vi "epx_Vector_SC_Menu.vi"(8 "Run Mode?":bool, 11 "MenuRef":refnum<k9>) -> ()   [LabVIEW 2011, in "NI_EP_Basic.lvlib" / "EPX Vector Diagram.xctl"]
uses:
  <vilib>/addons/Electrical Power/Basic/Controls/Vector Diagram/EPX Vector Diagram.xctl
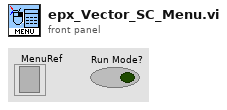
[diagram p1: front panel]
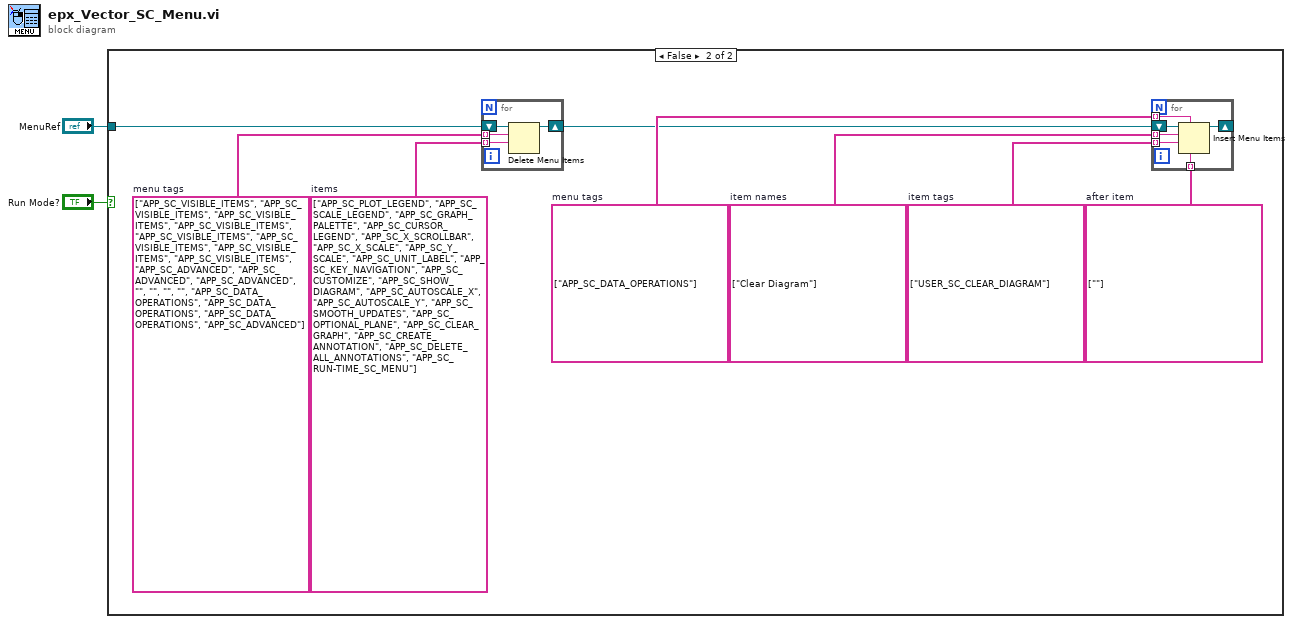
[diagram p0: block diagram]
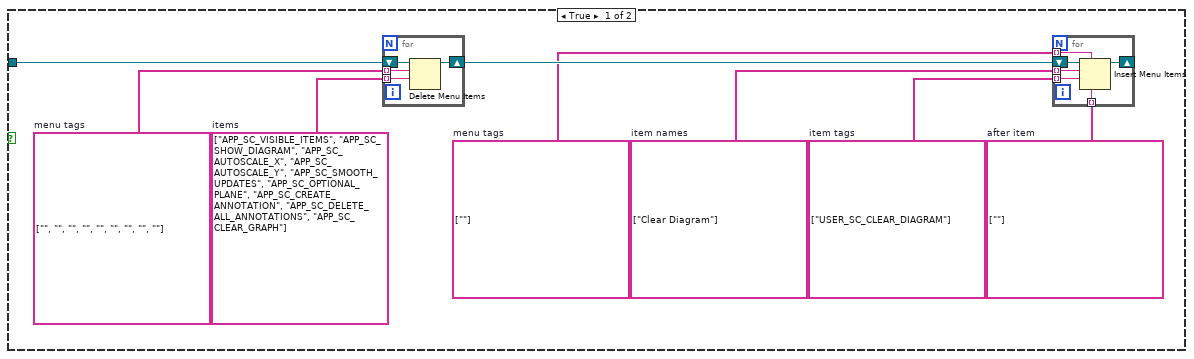
[diagram p2: hidden frame]
diagram:
  n1 = case shown="False" "Run Mode?" {
    tunnel: "MenuRef" -> [w10 w28]
    frame True {
      w3 = string[] [""]  # menu tags
      w4 = string[] ["Clear Diagram"]  # item names
      w5 = string[] ["USER_SC_CLEAR_DIAGRAM"]  # item tags
      w6 = string[] [""]  # after item
      w9 = string[] ["", "", "", "", "", "", "", "", ""]  # menu tags
      w8 = string[] ["APP_SC_VISIBLE_ITEMS", "APP_SC_SHOW_DIAGRAM", "APP_SC_AUTOSCALE_X", "APP_SC_AUTOSCALE_Y", "APP_SC_SMOOTH_UPDATES", "APP_SC_OPTIONAL_PLANE", "APP_SC_CREATE_ANNOTATION", "APP_SC_DELETE_ALL_ANNOTATIONS", "APP_SC_CLEAR_GRAPH"]  # items
      n2 = for {
        tunnel: w8 -> [w19] mode=indexing
        tunnel: w9 -> [w18] mode=indexing
        shift-right: [w17] -> w7
        shift-left: w10 -> [w20]
        n3 = Delete Menu Items(7:w19, 8:w18, 9:w20) -> (3:w17:refnum<k9>)  [unwired: 1 in, 1 out]
      }
      n4 = for {
        tunnel: w5 -> [w15] mode=indexing
        tunnel: w4 -> [w14] mode=indexing
        shift-right: [w13] -> _
        shift-left: w7 -> [w16]
        tunnel: w6 -> [w12] mode=indexing
        tunnel: w3 -> [w11] mode=indexing
        n5 = Insert Menu Items(4:w12, 5:w11, 7:w15, 8:w14, 9:w16) -> (3:w13:refnum<k9>)  [unwired: 1 in, 2 out]
      }
    }
    frame False {
      w22 = string[] ["APP_SC_DATA_OPERATIONS"]  # menu tags
      w23 = string[] ["Clear Diagram"]  # item names
      w24 = string[] ["USER_SC_CLEAR_DIAGRAM"]  # item tags
      w25 = string[] [""]  # after item
      w27 = string[] ["APP_SC_VISIBLE_ITEMS", "APP_SC_VISIBLE_ITEMS", "APP_SC_VISIBLE_ITEMS", "APP_SC_VISIBLE_ITEMS", "APP_SC_VISIBLE_ITEMS", "APP_SC_VISIBLE_ITEMS", "APP_SC_VISIBLE_ITEMS", "APP_SC_VISIBLE_ITEMS", "APP_SC_ADVANCED", "APP_SC_ADVANCED", "APP_SC_ADVANCED", "", "", "", "", "APP_SC_DATA_OPERATIONS", "APP_SC_DATA_OPERATIONS", "APP_SC_DATA_OPERATIONS", "APP_SC_ADVANCED"]  # menu tags
      w26 = string[] ["APP_SC_PLOT_LEGEND", "APP_SC_SCALE_LEGEND", "APP_SC_GRAPH_PALETTE", "APP_SC_CURSOR_LEGEND", "APP_SC_X_SCROLLBAR", "APP_SC_X_SCALE", "APP_SC_Y_SCALE", "APP_SC_UNIT_LABEL", "APP_SC_KEY_NAVIGATION", "APP_SC_CUSTOMIZE", "APP_SC_SHOW_DIAGRAM", "APP_SC_AUTOSCALE_X", "APP_SC_AUTOSCALE_Y", "APP_SC_SMOOTH_UPDATES", "APP_SC_OPTIONAL_PLANE", "APP_SC_CLEAR_GRAPH", "APP_SC_CREATE_ANNOTATION", "APP_SC_DELETE_ALL_ANNOTATIONS", "APP_SC_RUN-TIME_SC_MENU"]  # items
      n6 = for {
        tunnel: w26 -> [w37] mode=indexing
        tunnel: w27 -> [w36] mode=indexing
        shift-right: [w35] -> w21
        shift-left: w28 -> [w38]
        n7 = Delete Menu Items(7:w37, 8:w36, 9:w38) -> (3:w35:refnum<k9>)  [unwired: 1 in, 1 out]
      }
      n8 = for {
        tunnel: w24 -> [w33] mode=indexing
        tunnel: w23 -> [w32] mode=indexing
        shift-right: [w31] -> _
        shift-left: w21 -> [w34]
        tunnel: w25 -> [w30] mode=indexing
        tunnel: w22 -> [w29] mode=indexing
        n9 = Insert Menu Items(4:w30, 5:w29, 7:w33, 8:w32, 9:w34) -> (3:w31:refnum<k9>)  [unwired: 1 in, 2 out]
      }
    }
  }
